vi "Example Write Read Type 2.vi"() -> ()   [LabVIEW 2010]
uses:
  C:/tf/play/labview/Tinkerforge.dll
panel:
  out "events":string
  in  "stop":bool
  in  "uid":string="ooK"
  in  "port":i32=4223
  in  "host":string="localhost"
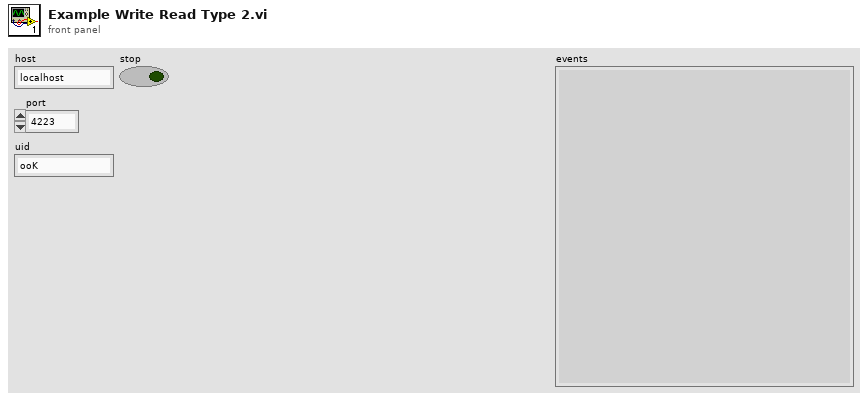
[diagram p1: front panel]
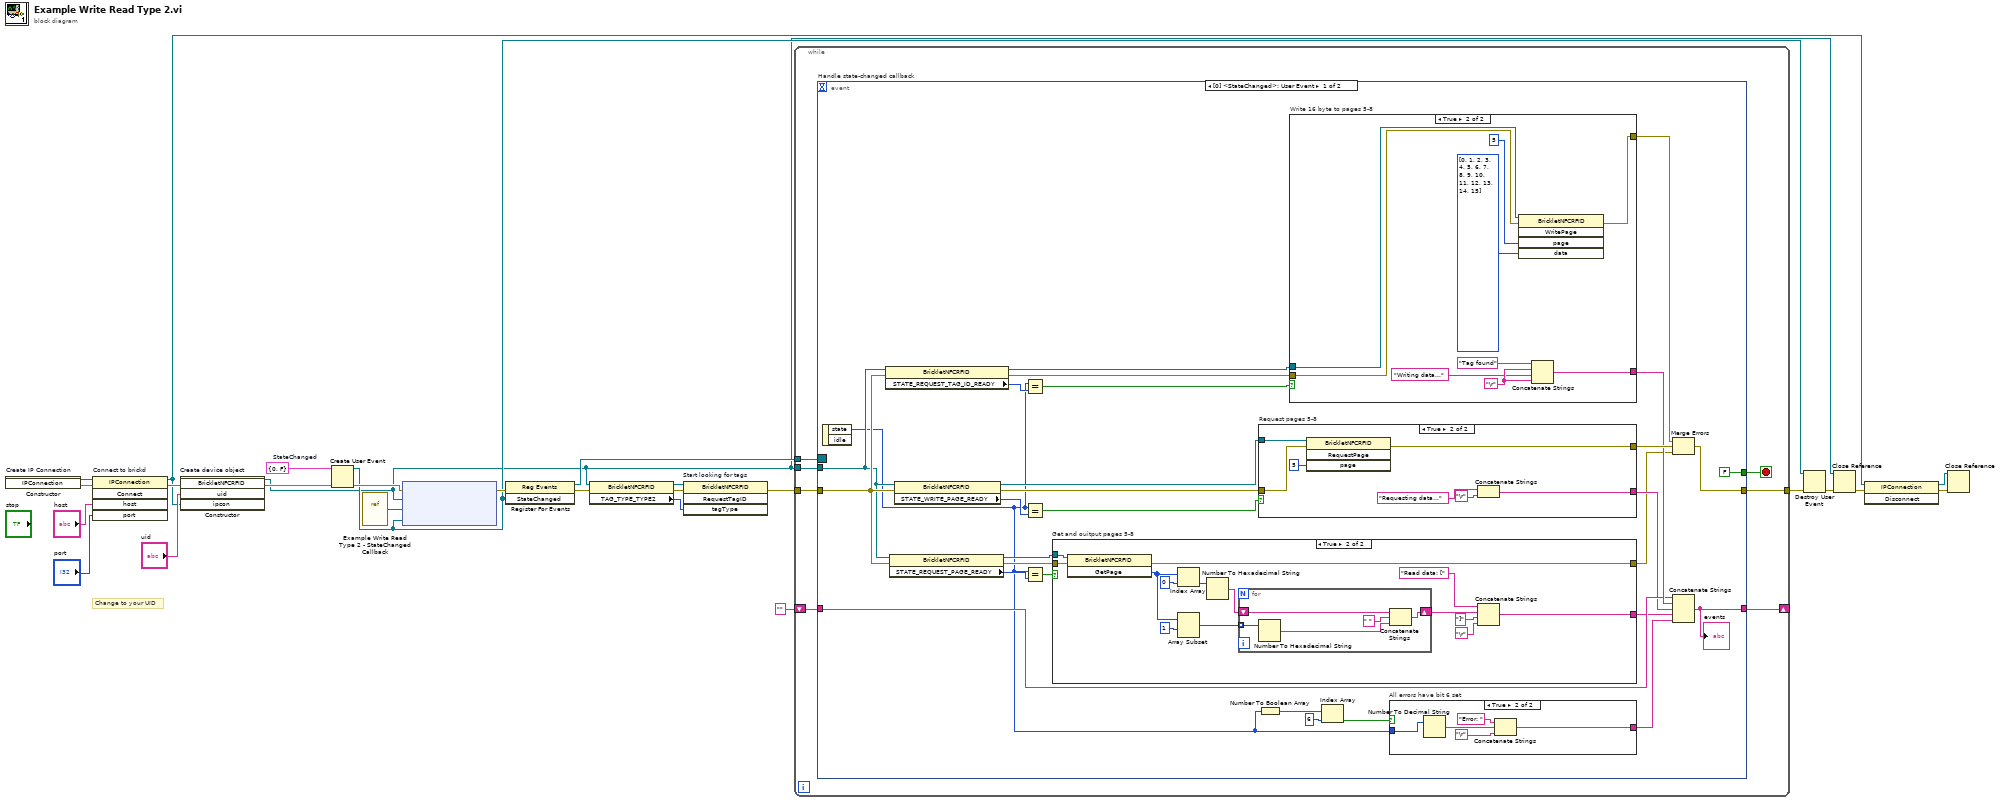
[diagram p0: block diagram]
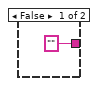
[diagram p2: hidden frame]
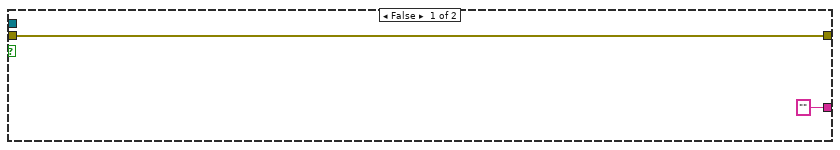
[diagram p3: hidden frame]
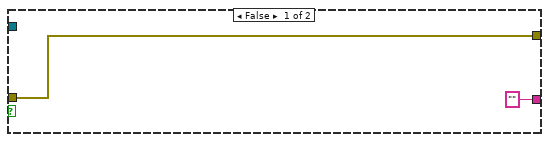
[diagram p4: hidden frame]
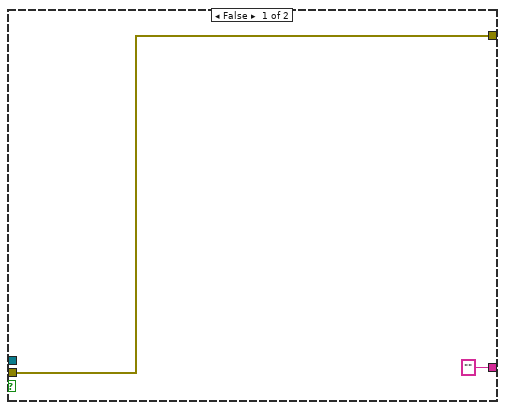
[diagram p5: hidden frame]
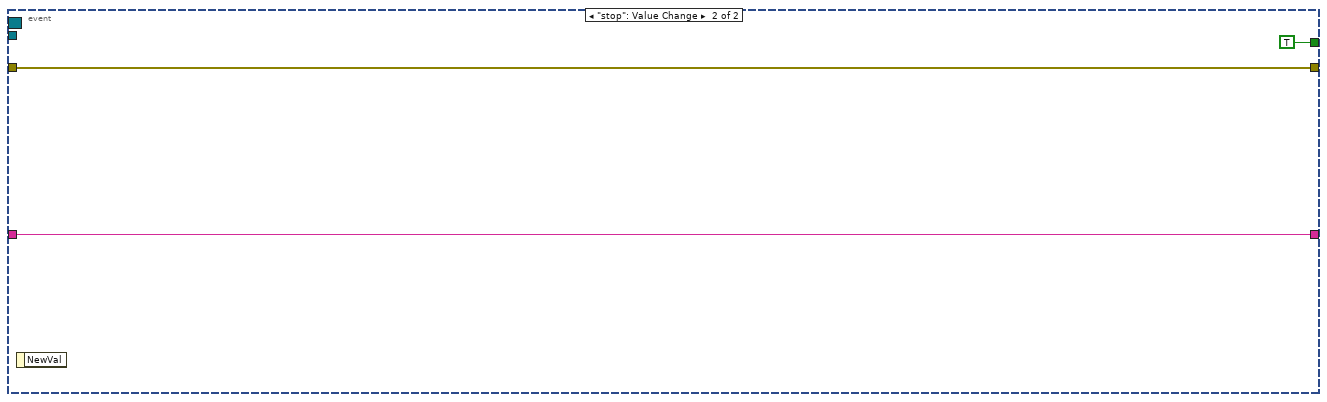
[diagram p6: hidden frame]
diagram:
  w11 = cluster{"state":u8, "idle":bool} {"state"=0, "idle"=FALSE}  # StateChanged
  # "Change to your UID"
  n1 = constructor on="Create IP Connection" class="IPConnection"() -> (reference out=w26:refnum<k24>, error out=w10:errorcluster)  [unwired: 3 in, 1 out]
  n2 = invoke on="Connect to brickd" class="IPConnection" method="Connect"(reference=w26, error in=w10, "host"="host", "port"="port") -> (reference out=w19:refnum<k24>, error out=w22:errorcluster)  [unwired: 1 in, 3 out]
  n3 = constructor on="Create device object" class="BrickletNFCRFID"(error in=w22, "uid"="uid", "ipcon"=w19) -> (reference out=w3:refnum<k24>, error out=w9:errorcluster)  [unwired: 2 in, 3 out]
  n4 = Create User Event(user event datatype=w11, error in=w9) -> (user event=w13:refnum<user-event>, error out=w17:errorcluster)
  n5 = vi-ref "Example Write Read Type 2 - StateChanged Callback.vi"() -> ("vi reference"=w1:refnum<vi>)
  n6 = node ("Register Event Callback")(w17, w3, w1, w13) -> (w16:errorcluster)  [unwired: 1 in, 1 out]
  n7 = register-events(error in=w16, w13) -> (reference out=w15:refnum<event-registration>, error out=w6:errorcluster)  [unwired: 1 in]
  n8 = property class="BrickletNFCRFID"(reference=w3, error in=w6) -> (reference out=w7:refnum<k24>, error out=w5:errorcluster, "TAG_TYPE_TYPE2"=w4:u8)
  n9 = invoke on="Start looking for tags" class="BrickletNFCRFID" method="RequestTagID"(reference=w7, error in=w5, "tagType"=w4) -> (error out=w8:errorcluster)  [unwired: 1 in, 3 out]
  n10 = while {
    tunnel: w15 -> [w33]
    tunnel: [w32] -> w14
    tunnel: w8 -> [w31]
    tunnel: w3 -> [w29]
    shift-right: [w27] -> _
    shift-left: "" -> [w28]
    stop <- w30 stop-if-true
    n11 = event "Handle state-changed callback" shown="[0] <StateChanged>: User Event" {
      selector: w33 -> [_ _]
      dyn-events: _ -> [_ _]
      timeout: _ -> [_ _]
      tunnel: [w52 w111] -> w32
      tunnel: w31 -> [w42 w111]
      tunnel: [FALSE TRUE] -> w30
      tunnel: w29 -> [w41 _]
      tunnel: w28 -> [w48 w110]
      tunnel: [w50 w110] -> w27
      event User Event {
        n12 = event-data() -> ("state"=w34:u8)  [unwired: 1 in, 1 out]
        n13 = property class="BrickletNFCRFID"(reference=w41, error in=w42) -> (reference out=w59:refnum<k24>, error out=w58:errorcluster, "STATE_REQUEST_TAG_ID_READY"=w61:u8)
        n14 = property class="BrickletNFCRFID"(reference=w41, error in=w42) -> (reference out=w44:refnum<k24>, error out=w43:errorcluster, "STATE_REQUEST_PAGE_READY"=w46:u8)
        n15 = property class="BrickletNFCRFID"(reference=w41, error in=w42) -> (reference out=w55:refnum<k24>, error out=w54:errorcluster, "STATE_WRITE_PAGE_READY"=w57:u8)
        n16 = Equal?(x=w34, y=w61) -> (x = y?=w60:bool)
        n17 = Equal?(x=w34, y=w57) -> (x = y?=w56:bool)
        n18 = Equal?(x=w34, y=w46) -> (x = y?=w45:bool)
        n19 = case "Get and ouitput pages 5-8" shown="True" w45 {
          tunnel: w44 -> [_ w84]
          tunnel: w43 -> [w70 w83]
          tunnel: [w70 w82] -> w37
          tunnel: ["" w80] -> w36
          frame False {
          }
          frame True {
            n20 = invoke class="BrickletNFCRFID" method="GetPage"(reference=w84, error in=w83) -> (error out=w82:errorcluster, "GetPage"=w75:u8[])  [unwired: 1 in, 1 out]
            n21 = Index Array(array=w75, index=0) -> (element=w76:u8)
            n22 = Array Subset(array=w75, index=1) -> (w73:u8[])  [unwired: 1 in]
            n23 = Number To Hexadecimal String(2:w76) -> (0:w72:string)  [unwired: 1 in]
            n24 = for {
              tunnel: w73 -> [w89] mode=indexing
              shift-right: [w85] -> w71
              shift-left: w72 -> [w88]
              n25 = Number To Hexadecimal String(2:w89) -> (0:w86:string)  [unwired: 1 in]
              n26 = Concatenate Strings(w88, " " ("string"), w86) -> (w85:string)
            }
            n27 = Concatenate Strings("Read data: [" ("string"), w71, "]", "\r") -> (w80:string)
          }
        }
        n28 = case "Request pages 5-8" shown="True" w56 {
          tunnel: w55 -> [_ w97]
          tunnel: w54 -> [w91 w96]
          tunnel: [w91 w95] -> w51
          tunnel: ["" w92] -> w47
          frame False {
          }
          frame True {
            n29 = invoke class="BrickletNFCRFID" method="RequestPage"(reference=w97, error in=w96, "page"=5) -> (error out=w95:errorcluster)  [unwired: 1 in, 3 out]
            n30 = Concatenate Strings("Requesting data..." ("string"), "\r") -> (w92:string)
          }
        }
        n31 = Number To Boolean Array(number=w34) -> (Boolean array=w40:bool[])
        n32 = case "Write 16 byte to pages 5-8" shown="True" w60 {
          tunnel: w59 -> [_ w109]
          tunnel: w58 -> [w100 w108]
          tunnel: [w100 w107] -> w53
          tunnel: ["" w101] -> w49
          frame False {
          }
          frame True {
            w103 = "\r"
            n33 = invoke class="BrickletNFCRFID" method="WritePage"(reference=w109, error in=w108, "page"=5, "data"=u8[] [0, 1, 2, 3, 4, 5, 6, 7, 8, 9, 10, 11, 12, 13, 14, 15]) -> (error out=w107:errorcluster)  [unwired: 1 in, 4 out]
            n34 = Concatenate Strings("Tag found", w103, "Writing data..." ("string"), w103) -> (w101:string)
          }
        }
        n35 = Index Array(array=w40, index=6) -> (element=w38:bool)
        n36 = case "All errors have bit 6 set" shown="True" w38 {
          tunnel: ["" w64] -> w35
          tunnel: w34 -> [_ w68]
          frame False {
          }
          frame True {
            n37 = Number To Decimal String(number=w68) -> (decimal integer string=w66:string)  [unwired: 1 in]
            n38 = Concatenate Strings("Error: ", w66, "\r") -> (w64:string)
          }
        }
        n39 = Merge Errors(w53, w51, w37) -> (w52:errorcluster)
        n40 = Concatenate Strings(w48, w49, w47, w36, w35) -> (w50:string)
        "events" <- w50
      }
      event "stop": Value Change {
        n41 = event-data() -> ()  [unwired: 1 in, 1 out]
      }
    }
  }
  n42 = Destroy User Event(user event=w13, error in=w14) -> (error out=w12:errorcluster)
  n43 = Close Reference(reference=w3, error in (no error)=w12) -> (error out=w21:errorcluster)
  n44 = invoke class="IPConnection" method="Disconnect"(reference=w19, error in=w21) -> (reference out=w18:refnum<k24>, error out=w20:errorcluster)  [unwired: 1 in, 1 out]
  n45 = Close Reference(reference=w18, error in (no error)=w20) -> ()  [unwired: 1 out]
